vi "CALC_Get_EMA_Coeffs.vi"(2 "EMA length":i32=11, 3 "alpha":dbl=0.3) -> (1 "EMA coeffs":dbl[](array[numeric]))   [LabVIEW 2018, in "Tracker.lvlib"]
uses:
  Tracker.lvlib
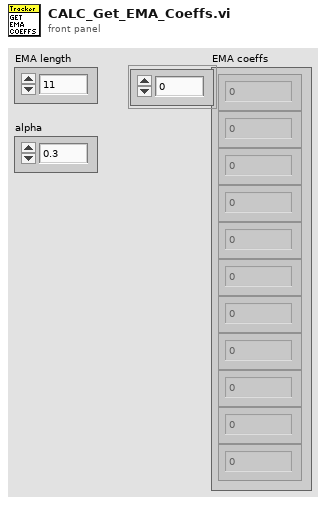
[diagram p1: front panel]
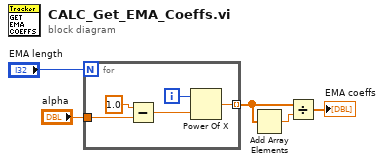
[diagram p0: block diagram]
diagram:
  n1 = for {
    N: "EMA length" -> [_]
    tunnel: "alpha" -> [w9]
    tunnel: [w6] -> w2 mode=indexing
    i -> [w7]
    n2 = Subtract(x=1.0, y=w9) -> (x-y=w8:dbl)
    n3 = Power Of X(1:w8, 2:w7) -> (0:w6:dbl)
  }
  n4 = Add Array Elements(numeric array=w2) -> (sum=w1:dbl)
  n5 = Divide(x=w2, y=w1) -> (x/y=→"EMA coeffs":dbl[])
